vi "Saturation.vi"   [LabVIEW 2017, in "NI_AdvCtrl_nonlinear.lvlib"]
doc: "LabVIEW no longer supports this VI. You can obtain similar functionality by installing the LabVIEW Simulation Module.\n\nLimits the valid range of a signal. The output point is equal to the upper limit, if input point>upper limit. The output point is equal to the lower limit, if input point<lower limit. In all other cases it is output point=input point."
uses:
  <vilib>/addons/control/advanced/NI_AdvCtrl_nonlinear.lvlib
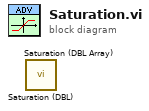
[diagram p0: block diagram]
diagram:
  n1 = call <vilib>:"Saturation (DBL).vi"() -> ()  [unwired: 4 in, 1 out]
  n2 = call <vilib>:"Saturation (DBL Array).vi"() -> ()  [unwired: 4 in, 1 out]
